vi "UpdateImg.vi"(7 "Enum":enum16{"Mark", "Clear All"}(ring), 8 "error in (no error)":errorcluster, 11 "EpiWrapper in":refnum<class "EpiWrapper.lvclass">) -> (0 "error out":errorcluster, 3 "EpiWrapper out":refnum<class "EpiWrapper.lvclass">)   [LabVIEW 2012, in "EpiWrapper.lvclass"]
uses:
  EpiWrapper.lvclass
  EpiWrapper.lvclass/EpiWrapper.ctl
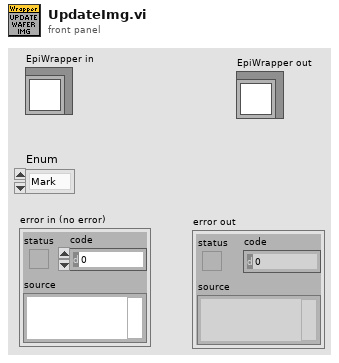
[diagram p1: front panel]
types:
  T1 = cluster{"Width":i16, "Style":enum32{"Solid", "Dash", "Dot", "DashDot", "DashDotDot"}}
  T2 = typedef "MeasureControl.ctl" = cluster{"Pass":bool, "Fail":bool, "Measure":bool, "Area":T3, "TestData":T4, "Graph":cluster{"Y":dbl[], "Y":dbl[]}[]}
  T3 = typedef "TestArea.ctl" = string
  T4 = typedef "TestData.ctl" = cluster{"20mA Data":cluster{"Area":string, "Current,mA":dbl, "Power":dbl, "WL":dbl, "Voltage":dbl, "Knee Current":dbl, "Reverse":dbl}, "50mA Data":cluster{"Area":string, "Current,mA":dbl, "Power":dbl, "WL":dbl, "Voltage":dbl}}
  T5 = typedef "MapPOS.ctl" = cluster{"Top":cluster{"left":i16, "top":i16, "right":i16, "bottom":i16}, "CenterC":cluster{"left":i16, "top":i16, "right":i16, "bottom":i16}, "CenterB":cluster{"left":i16, "top":i16, "right":i16, "bottom":i16}, "CenterA":cluster{"left":i16, "top":i16, "right":i16, "bottom":i16}, "Left":cluster{"left":i16, "top":i16, "right":i16, "bottom":i16}, "Right":cluster{"left":i16, "top":i16, "right":i16, "bottom":i16}}
  T6 = cluster{"left":i16, "top":i16, "right":i16, "bottom":i16}[]
  T7 = typedef "Waferimage.ctl" = picture
  T8 = cluster{"left":i16, "top":i16, "right":i16, "bottom":i16}
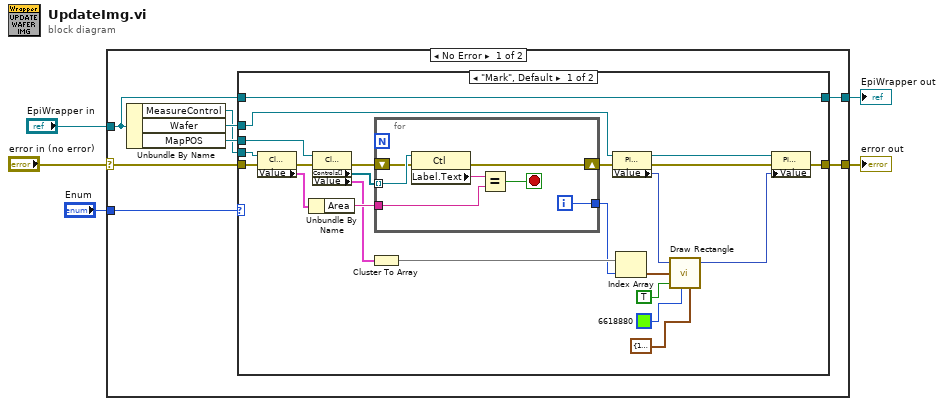
[diagram p0: block diagram]
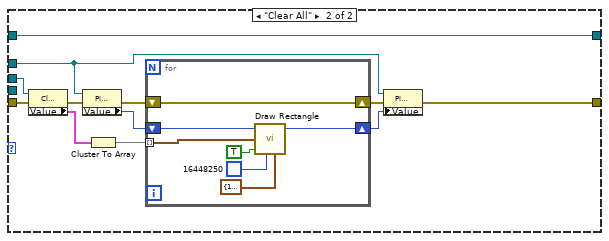
[diagram p2: hidden frame]
diagram:
  n1 = case shown="No Error" "error in (no error)" {
    selector: "error in (no error)" -> [w11 w64]
    tunnel: [w9 w64] -> w4
    tunnel: [w6 w63] -> w2
    tunnel: "EpiWrapper in" -> [w7 w63]
    tunnel: "Enum" -> [w8 _]
    frame No Error {
      n2 = Unbundle By Name(w7) -> ("MeasureControl"=w10:refnum<vi>, "Wafer"=w13:refnum<vi>, "MapPOS"=w12:refnum<vi>)
      n3 = case shown="\"Mark\", Default" w8 {
        tunnel: w13 -> [w24 w44]
        tunnel: w12 -> [w23 w54]
        tunnel: w11 -> [w20 w49]
        tunnel: w10 -> [w19 _]
        tunnel: [w16 w55] -> w9
        tunnel: w7 -> [w15 w46]
        tunnel: [w15 w46] -> w6
        frame "Mark", Default {
          n4 = property class="Clust (strict)"(reference=w19, error in=w20) -> (error out=w21:errorcluster, "Value"=w35:T2)  [unwired: 1 out]
          n5 = Unbundle By Name(w35) -> ("Area"=w36:T3)
          n6 = property class="Clust (strict)"(reference=w23, error in=w21) -> (error out=w22:errorcluster, "Controls[]"=w25:refnum<vi>[], "Value"=w31:T5)  [unwired: 1 out]
          n7 = Cluster To Array(cluster=w31) -> (array=w27:T6)
          n8 = for {
            tunnel: w25 -> [w43] mode=indexing
            tunnel: [w40] -> w26
            shift-right: [w38] -> w18
            shift-left: w22 -> [w39]
            tunnel: w36 -> [w37]
            i -> [w40]
            stop <- w41 stop-if-true
            n9 = property class="Ctl"(reference=w43, error in=w39) -> (error out=w38:errorcluster, "Label.Text"=w42:string)  [unwired: 1 out]
            n10 = Equal?(x=w42, y=w37) -> (x = y?=w41:bool)
          }
          n11 = property class="Pict (strict)"(reference=w24, error in=w18) -> (reference out=w33:refnum<vi>, error out=w17:errorcluster, "Value"=w32:T7)
          n12 = Index Array(array=w27, index=w26) -> (element=w28:T8)
          n13 = call <vilib>:"Draw Rectangle.vi"("picture"=w32, "rect"=w28, "fill?(F)"=TRUE, "color(black)"=u32 6618880, "pen"=T1 {"Width"=1, "Style"=enum."Solid"}) -> ("new picture"=w34:picture)  [unwired: 4 in]
          n14 = property class="Pict (strict)"(reference=w33, error in=w17, "Value"=w34) -> (error out=w16:errorcluster)  [unwired: 1 out]
        }
        frame "Clear All" {
          n15 = property class="Clust (strict)"(reference=w54, error in=w49) -> (error out=w52:errorcluster, "Value"=w53:T5)  [unwired: 1 out]
          n16 = property class="Pict (strict)"(reference=w44, error in=w52) -> (error out=w48:errorcluster, "Value"=w51:T7)  [unwired: 1 out]
          n17 = Cluster To Array(cluster=w53) -> (array=w50:T6)
          n18 = for {
            shift-right: [w58] -> w45
            shift-left: w51 -> [w59]
            tunnel: w50 -> [w57] mode=indexing
            shift-right: [w56] -> w47
            shift-left: w48 -> [w56]
            n19 = call <vilib>:"Draw Rectangle.vi"("picture"=w59, "rect"=w57, "fill?(F)"=TRUE, "color(black)"=u32 16448250, "pen"=T1 {"Width"=1, "Style"=enum."Solid"}) -> ("new picture"=w58:picture)  [unwired: 4 in]
          }
          n20 = property class="Pict (strict)"(reference=w44, error in=w47, "Value"=w45) -> (error out=w55:errorcluster)  [unwired: 1 out]
        }
      }
    }
    frame Error {
    }
  }
  "error out" <- w4
  "EpiWrapper out" <- w2
